vi "SCD - Write FITS File.vi"(0 "A":i32[][](array[numeric]), 1 "FITS Header":T3={"Wavelength (nm)"=530.15, "Exposure (s)"=0.05, "Tuning Delay (ms)"=1000.0, "Beam Type (-1/1)"=1.0, "Tuning Voltages"=[1.111, 2.222, 3.333, 4.444], "Observer"="observer", "Light Shapping Diffuser"=enum."In Beam", "Comment"="", "Data Type"=9, "Mod Cycles"=0, "SCD Calibration Optics"=enum."1 - Polarizer @0, I+Q", "SCD Emission Line Filter"=enum."1-557.6nm", "Cookbook"="", "COMP-S Calibration Wheel"=enum."Dark", "COMP-S Andover Filter Wheel"=enum."530.3nm/HWB 0.34nm (Fe XIV)", "FOV Rotation (deg)"=66.0, "Objective Lens Position (mm)"=0.0, "Occulter size"=0.0, "Time End"=timestamp(3382374145.421875 s since 1904-01-01), "Acc Exposure (s)"=0.0, "Time Stamp Array"=[], "Camera Serial Number"=[], "Camera Temp"=[], "Camera PI (mm)"=[0.0, 0.0, 0.0], "Time Start"=timestamp(3382374145.421875 s since 1904-01-01), "Peripherals"={"ILX controler"=FALSE, "Zone temperatures"=FALSE, "Andor"=FALSE, "Andor 2"=FALSE, "PI Stages"=FALSE, "AISAS mechanisms"=FALSE, "AISAS Mech.lvclass"=refnum, "Zone temp ref"=variant, "FWs"=FALSE}, "FITS paths"=[path " ", path " ", path " ", path " "], "Cameras"=enum."Andor", "load preset cbk"=FALSE, "periodic check count"=0} {"Camera PI (mm)" format="%_3g"; "Acc Exposure (s)" format="%^.3g"; "Occulter size" format="%.2f"; "Objective Lens Position (mm)" min=70.0 max=152.0 format="%.2f"; "FOV Rotation (deg)" format="%.1f"; "Data Type" items=["LIVE", "DARK", "FLAT", "CALI", "OBSE", "ABSO", "AURE", "TARG", "OBJE", "HOLE", "OREX", "THRO", "CHIP"]; "Exposure (s)" format="%^.3g"; "Wavelength (nm)" format="%_6g"}, 2 "Neo Info":T1={"Handle"=104, "Pixel Encoding"="Mono16", "AOI Width"=2560, "AOI Height"=2160, "AOI Stride"=5136, "Image Bytes"=11098896, "Image Pixels"=5529600, "Row Readout Time"=9.371428571428572e-06, "Frame Readout Time"=0.010121142857142858, "Interframe Time"=8.434285714285715e-05, "Semaphore"=refnum, "SerialNumber"="SCC-02209", "Camera Model"="DC-152Q-C00-FI", "Controller ID"="3", "Firmware Version"="13.8.26.122", "Shutter"="Global", "Binning"=0, "Time at Synch"=timestamp(3029526000.379448 s since 1904-01-01), "Idx"=0} {"Time at Synch" format="%<%H:%M:%S>T"; "Interframe Time" format="%#_3g"; "Frame Readout Time" format="%_3g"; "Row Readout Time" format="%_3g"}, 5 "B":i32[][](array[numeric]), 7 "C":i32[][](array[numeric]), 9 "D":i32[][](array[numeric]), 11 "error in":errorcluster, 12 "Image #":i32) -> (4 "FITS Path Out":path=path "G:/SCD Data/Level-0/20141030/20141030.160747.FTS", 6 "<ADU>":dbl[](array[numeric]), 15 "error out":errorcluster)   [LabVIEW 2014]
doc: "Use this template to build a VI to use as a subVI."
uses:
  AISAS/Controls/Diffuser.ctl
  Controls/SCD - Calibration Optics Filter Wheel.ctl
  Controls/SCD - EDT - Emission Line Filter Wheel.ctl
  Controls/SCD - FITS Cluster.ctl
  Camera/Andor Neo Info.ctl
  Controls/CoMP-S Controls/Polarization Optics Filter Wheel.ctl
  Controls/CoMP-S Controls/Emission Line Filter Wheel.ctl
  AISAS/Controls/focus.ctl
  AISAS/Mech/AISAS Mech.lvclass
  Controls/peripherals.ctl
  Controls/Cameras select.ctl
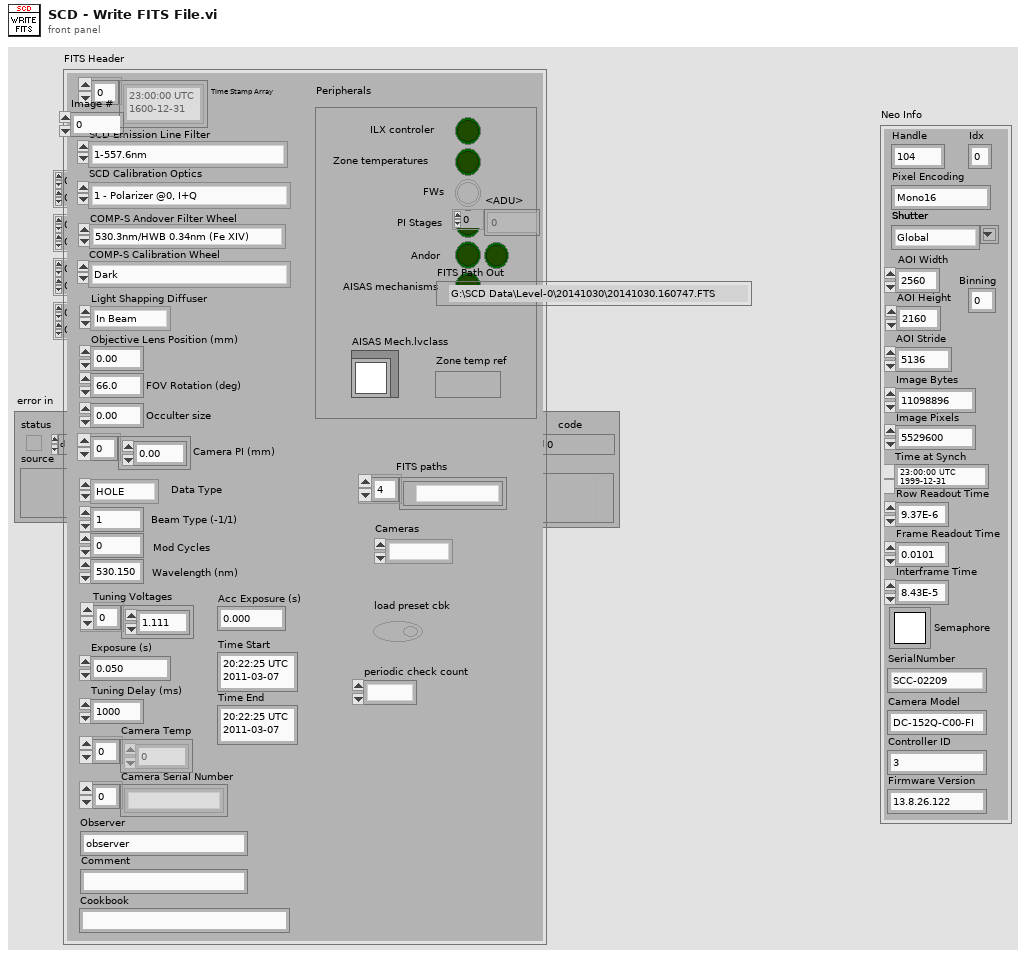
[diagram p1: front panel]
types:
  T1 = typedef "Andor Neo Info.ctl" = cluster{"Handle":i32, "Pixel Encoding":string, "AOI Width":i64, "AOI Height":i64, "AOI Stride":i64, "Image Bytes":i64, "Image Pixels":i64, "Row Readout Time":dbl, "Frame Readout Time":dbl, "Interframe Time":dbl, "Semaphore":T2, "SerialNumber":string, "Camera Model":string, "Controller ID":string, "Firmware Version":string, "Shutter":string, "Binning":u8, "Time at Synch":timestamp, "Idx":i32}
  T2 = typedef "Semaphore RefNum" = refnum<k1>
  T3 = typedef "SCD - FITS Cluster.ctl" = cluster{"Wavelength (nm)":dbl, "Exposure (s)":dbl, "Tuning Delay (ms)":dbl, "Beam Type (-1/1)":dbl, "Tuning Voltages":dbl[], "Observer":string, "Light Shapping Diffuser":T4, "Comment":string, "Data Type":u16, "Mod Cycles":u16, "SCD Calibration Optics":T5, "SCD Emission Line Filter":T6, "Cookbook":string, "COMP-S Calibration Wheel":T7, "COMP-S Andover Filter Wheel":T8, "FOV Rotation (deg)":dbl, "Objective Lens Position (mm)":T9, "Occulter size":dbl, "Time End":timestamp, "Acc Exposure (s)":dbl, "Time Stamp Array":timestamp[], "Camera Serial Number":string[], "Camera Temp":dbl[], "Camera PI (mm)":dbl[], "Time Start":timestamp, "Peripherals":T10, "FITS paths":path[], "Cameras":T11, "load preset cbk":bool, "periodic check count":i32}
  T4 = typedef "Diffuser.ctl" = enum16{"Out of Beam", "In Beam"}
  T5 = typedef "SCD - Calibration Optics Filter Wheel.ctl" = enum16{"1 - Polarizer @0, I+Q", "2 - Polarizer @90, I-Q", "3 - Polarizer @45, I+U", "4 - Polarizer @135, I-U", "5 - Polarizer @0, Retarder @45, I+V", "6 - Polarizer @0, Retarder @135, I-V", "7 - Dark", "8 - Clear", "9 - N/A"}
  T6 = typedef "SCD - EDT - Emission Line Filter Wheel.ctl" = enum16{"1-557.6nm", "2-587.6nm", "3-589.6nm", "4-630.2nm", "5-656.4nm", "6-849.8nm", "7-854.2nm", "8-866.2nm", "9-1083.0nm"}
  T7 = typedef "Polarization Optics Filter Wheel.ctl" = enum16{"Dark", "Clear", "Exchange Lens", "Polarizer @0, I+Q", "Polarizer @90, I-Q", "Polarizer @45, I+U", "Polarizer @135, I-U", "Polarizer @0, Retarder @45, I+V", "Polarizer @0, Retarder @135, I-V"}
  T8 = typedef "Emission Line Filter Wheel.ctl" = enum16{"530.3nm/HWB 0.34nm (Fe XIV)", "587.6nm/HBW 0.44nm (He I D3)", "637.5nm/HBW 0.53nm (Fe X)", "656.3nm/HBW 0.57nm (H-Alpha)", "789.2nm/HBW 0.85nm (Fe XI)", "854.2nm/HBW 1.01nm (Ca I)", "1074.7nm/HBW 2.34nm (Fe XIII)", "1079.8nm/HBW 1.64nm (Fe XIII)", "1083.0nm/HBW 1.66nm (He I)"}
  T9 = typedef "focus.ctl" = dbl
  T10 = typedef "peripherals.ctl" = cluster{"ILX controler":bool, "Zone temperatures":bool, "Andor":bool, "Andor 2":bool, "PI Stages":bool, "AISAS mechanisms":bool, "AISAS Mech.lvclass":refnum<class "AISAS Mech.lvclass">, "Zone temp ref":variant, "FWs":bool}
  T11 = typedef "Cameras select.ctl" = enum16{"Andor", "GDR"}
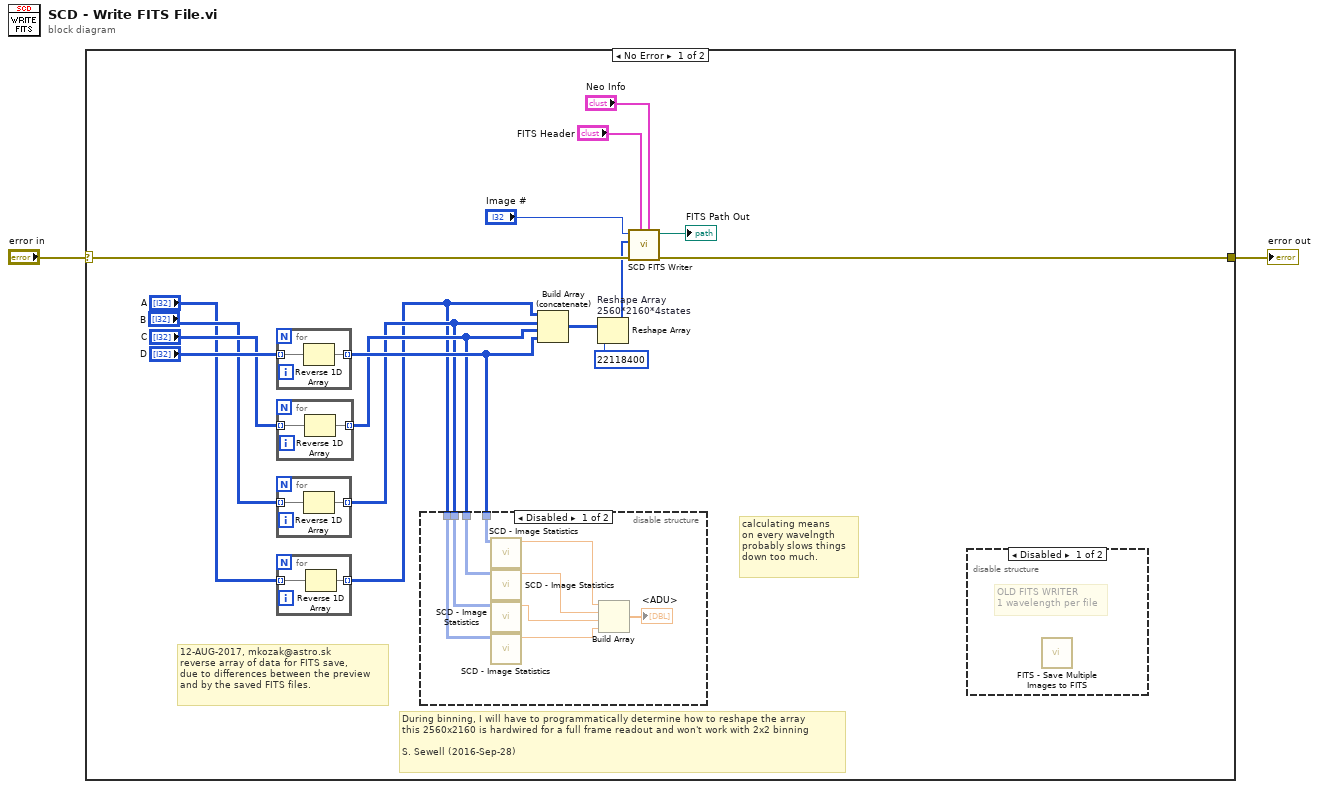
[diagram p0: block diagram]
diagram:
  n1 = case shown="No Error" "error in" {
    selector: "error in" -> [w17 w37]
    tunnel: [w15 w37] -> w1
    frame No Error {
      # "12-AUG-2017, mkozak@astro.sk\nreverse array of data for FITS save, \ndue to differences between the preview\nand by the saved FITS files."
      # "calculating means\non every wavelngth\nprobably slows things\ndown too much."
      # "During binning, I will have to programmatically determine how to reshape the array\nthis 2560x2160 is hardwired for a full frame readout and won't work with 2x2 binning\n\nS. Sewell (2016-Sep-28)"
      n2 = for {
        tunnel: "D" -> [w21] mode=indexing
        tunnel: [w20] -> w9 mode=indexing
        n3 = Reverse 1D Array(array=w21) -> (reversed array=w20:i32[])
      }
      n4 = for {
        tunnel: "C" -> [w27] mode=indexing
        tunnel: [w26] -> w7 mode=indexing
        n5 = Reverse 1D Array(array=w27) -> (reversed array=w26:i32[])
      }
      n6 = for {
        tunnel: "B" -> [w25] mode=indexing
        tunnel: [w24] -> w5 mode=indexing
        n7 = Reverse 1D Array(array=w25) -> (reversed array=w24:i32[])
      }
      n8 = for {
        tunnel: "A" -> [w23] mode=indexing
        tunnel: [w22] -> w3 mode=indexing
        n9 = Reverse 1D Array(array=w23) -> (reversed array=w22:i32[])
      }
      n10 = disable-structure shown="Disabled" {
        disable-tunnel: w3 -> [w36 _]
        disable-tunnel: w5 -> [w35 _]
        disable-tunnel: w9 -> [w34 _]
        disable-tunnel: w7 -> [w33 _]
        frame Disabled {
          n11 = call "SCD - Image Statistics.vi"("I32 Image"=w34) -> ("mean"=w32:dbl)  [unwired: 9 in, 1 out]
          n12 = call "SCD - Image Statistics.vi"("I32 Image"=w33) -> ("mean"=w31:dbl)  [unwired: 9 in, 1 out]
          n13 = call "SCD - Image Statistics.vi"("I32 Image"=w35) -> ("mean"=w30:dbl)  [unwired: 9 in, 1 out]
          n14 = call "SCD - Image Statistics.vi"("I32 Image"=w36) -> ("mean"=w29:dbl)  [unwired: 9 in, 1 out]
          n15 = Build Array(w32, w31, w30, w29) -> (→"<ADU>":dbl[])
        }
        frame Enabled {
        }
      }
      n16 = Build Array (concatenate)(w3, w5, w7, w9) -> (w18:i32[][])
      n17 = Reshape Array "Reshape Array\n2560*2160*4states"(w18, 22118400 ("dimension size")) -> (w11:i32[])
      n18 = call "SCD FITS Writer.vi"("Andor Neo Cluster"="Neo Info", "SCD FITS Cluster"="FITS Header", "error in"=w17, "Image Vector"=w11, "Wavelength (0..n)"="Image #") -> ("error out"=w15:errorcluster, "Current FITS Path"=→"FITS Path Out":path)  [unwired: 5 in]
      n19 = disable-structure shown="Disabled" {
        frame Disabled {
          # "OLD FITS WRITER\n1 wavelength per file"
          n20 = call "FITS - Save Multiple Images to FITS.vi"() -> ()  [unwired: 9 in, 3 out]
        }
        frame Enabled {
        }
      }
    }
    frame Error {
    }
  }
  "error out" <- w1
